vi "Read Flattened Buffer Configuration.vi"(8 "error in (no error)":errorcluster, 11 "CIF_CIPC_Chn in":refnum<class "CIF_CIPC_Chn.lvclass">) -> (0 "error out":errorcluster, 2 "Flattened Configuration":u8[](array[numeric]) format="%.0x", 3 "CIF_CIPC_Chn out":refnum<class "CIF_CIPC_Chn.lvclass">)   [LabVIEW 2021, in "CIF_CIPC_Chn.lvclass"]
uses:
  CIF_CIPC_Chn.lvclass
  CIF_CIPC_Chn.lvclass/CIF_CIPC_Chn.ctl
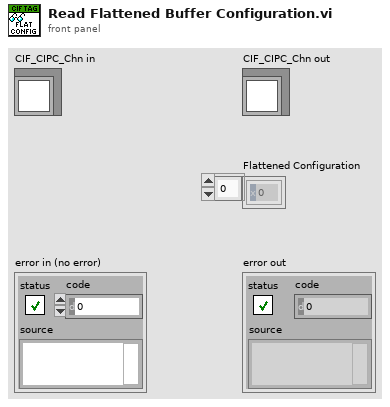
[diagram p1: front panel]
types:
  T1 = typedef "CIF_CIPC_Chn.lvclass/Buffer Configuration Data.ctl" = cluster{"Total Size":u32, "Read Size":u32, "Read Offset":u32, "CIPC BP References":T2, "Override CIPC Name":string, "Encoder Data":string}
  T2 = typedef "CIF_NI_CIPC.lvlib/Backpressure References.ctl" = cluster{"CIPC Reference":u64, "CIPC BP Reference":u64}
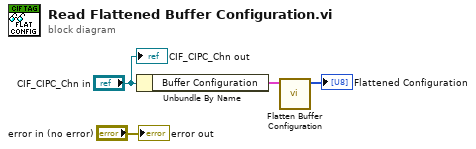
[diagram p0: block diagram]
diagram:
  n1 = Unbundle By Name("CIF_CIPC_Chn in") -> ("Buffer Configuration"=w2:T1)
  n2 = call "Flatten Buffer Configuration.vi"("Buffer Configuration"=w2) -> ("Flattened Configuration"=→"Flattened Configuration":u8[])  [unwired: 10 in]
  "error out" <- "error in (no error)"
  "CIF_CIPC_Chn out" <- "CIF_CIPC_Chn in"
